vi "FGV SUBVI.vi"(7 "Enum":enum16{"Get Data", "Set Data"}(ring), 11 "Data Input in":dbl) -> (3 "Data Input out":dbl)   [LabVIEW 2022 SP3]
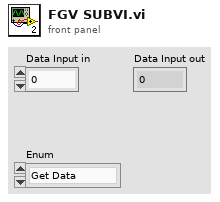
[diagram p1: front panel]
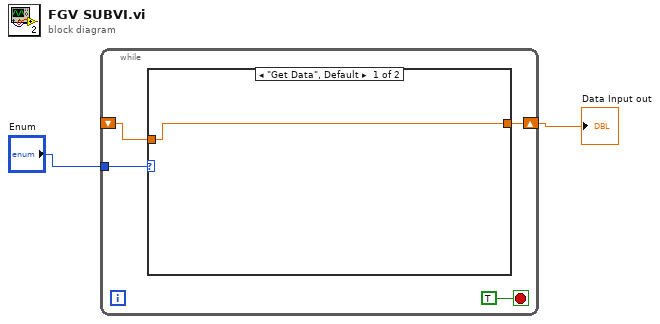
[diagram p0: block diagram]
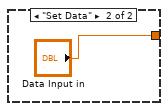
[diagram p2: hidden frame]
diagram:
  n1 = while {
    tunnel: "Enum" -> [w5]
    shift-right: [w3] -> w2
    shift-left: _ -> [w4]
    stop <- TRUE stop-if-true
    n2 = case shown="\"Get Data\", Default" w5 {
      tunnel: w4 -> [w7 _]
      tunnel: [w7 "Data Input in"] -> w3
      frame "Get Data", Default {
      }
      frame "Set Data" {
      }
    }
  }
  "Data Input out" <- w2
